vi "Data to Stage Request Status.vi"(1 "Data":u8[](array[numeric])) -> (0 "Stage Request Status":T1)   [LabVIEW 2016]
uses:
  Stage Request Status.ctl
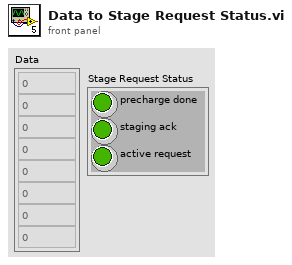
[diagram p1: front panel]
types:
  T1 = typedef "Stage Request Status.ctl" = cluster{"precharge done":bool, "staging ack":bool, "active request":bool}
  T2 = cluster{"[0]":bool, "[1]":bool, "[2]":bool, "[3]":bool, "[4]":bool, "[5]":bool, "[6]":bool}
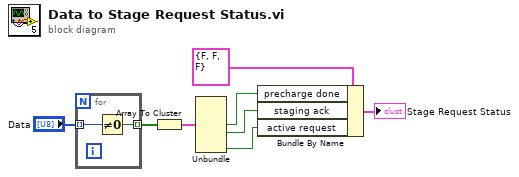
[diagram p0: block diagram]
diagram:
  n1 = for {
    tunnel: "Data" -> [w10] mode=indexing
    tunnel: [w9] -> w7 mode=indexing
    n2 = Not Equal To 0?(x=w10) -> (x != 0?=w9:bool)
  }
  n3 = Array To Cluster(array=w7) -> (cluster=w6:T2)
  n4 = Unbundle(w6) -> ("[3]"=w5:bool, "[4]"=w4:bool, "[6]"=w3:bool)  [unwired: 4 out]
  n5 = Bundle By Name(cluster=T1 {"precharge done"=FALSE, "staging ack"=FALSE, "active request"=FALSE} ("Stage Request Status"), "precharge done"=w5, "staging ack"=w4, "active request"=w3) -> (→"Stage Request Status":T1)
